vi "Update Simulated Instruments 4.1 to 4.2.vi"(2 "Instrument Information":T1) -> (7 "updated Instrument":T1)   [LabVIEW 2011]
uses:
  Instrument Record.ctl
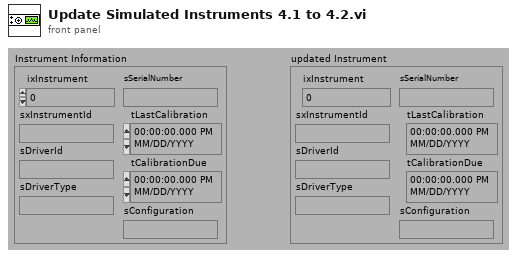
[diagram p1: front panel]
types:
  T1 = typedef "Instrument Record.ctl" = cluster{"ixInstrument":i32, "sxInstrumentId":string, "sDriverId":string, "sDriverType":string, "sSerialNumber":string, "tLastCalibration":timestamp, "tCalibrationDue":timestamp, "sConfiguration":string}
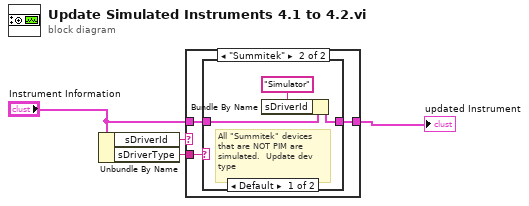
[diagram p0: block diagram]
diagram:
  n1 = Unbundle By Name("Instrument Information") -> ("sDriverId"=w4:string, "sDriverType"=w3:string)
  n2 = case shown="\"Summitek\"" w4 {
    tunnel: "Instrument Information" -> [w5 w7]
    tunnel: [w5 w6] -> w1
    tunnel: w3 -> [_ w8]
    frame Default {
    }
    frame "Summitek" {
      n3 = case shown="Default" w8 {
        tunnel: w7 -> [w11 w12]
        tunnel: [w10 w12] -> w6
        frame Default {
          # "All \"Summitek\" devices\nthat are NOT PIM are\nsimulated.  Update dev\ntype"
          n4 = Bundle By Name(cluster=w11, "sDriverId"="Simulator" ("Driver_ID")) -> (w10:T1)
        }
        frame "PIM" {
        }
      }
    }
  }
  "updated Instrument" <- w1
